vi "Packet Format.vi"(8 "error in":errorcluster, 11 "value":path) -> (0 "error out":errorcluster, 3 "data":T1(array[cluster]))   [LabVIEW 2014, in "Network Actor Library.lvlib" / "Network Actor.lvclass"]
uses:
  Network Actor.lvclass
  <vilib>/NI/GXML/_subVIs/GXML SearchParser/Search Parser.vi
  <vilib>/NI/GXML/GXML.lvlib
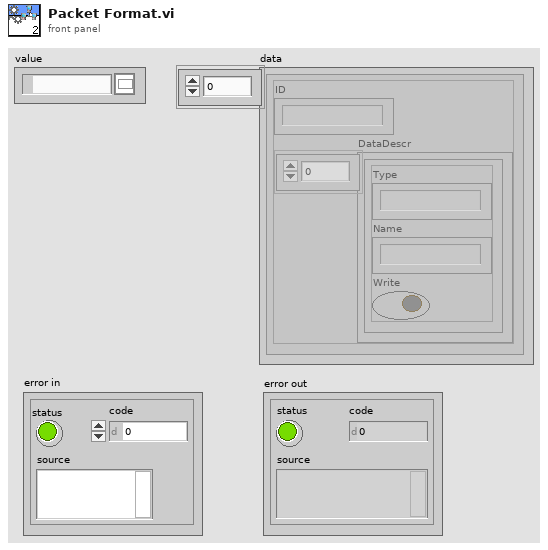
[diagram p1: front panel]
types:
  T1 = cluster{"ID":string, "DataDescr":cluster{"Type":string, "Name":string, "Write":bool}[]}[]
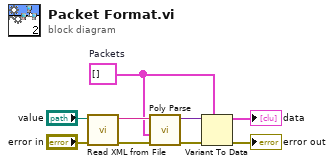
[diagram p0: block diagram]
diagram:
  w3 = T1 []  # Packets
  n1 = call <vilib>:"Read XML from File.vi"("error in"="error in", "XML File Path"="value") -> ("error out"=w6:errorcluster, "XML String Out"=w5:string)  [unwired: 8 in]
  n2 = call-poly <vilib>:"Poly Parse.vi"("error in"=w6, "TypeDesc"=w3, "XML String In"=w5) -> ("error out"=w8:errorcluster, "Parsed Data"=w7:variant)  [unwired: 7 in]
  n3 = Variant To Data(error in=w8, type=w3, Variant=w7) -> (data=→"data":T1, error out=→"error out":errorcluster)
